vi "HIS.vi"(0 "System no.":i32=1 min=1 max=4 step=1, 2 "DeviceID":i32[](array[numeric]), 3 "Property":i32[](array[numeric]), 5 "error in":errorcluster, 6 "ItemID":i32[](array[numeric]), 10 "Value":string[](array[string])) -> (14 "Controller error":bool, 19 "error out":errorcluster)   [LabVIEW 2026]
doc: "This VI sets values for items of human interface devices (HID). The VI waits 100 ms and queries ERR?. Properties can be colors, the blink time of a LED, the frequency of a force-feed back function, display text etc. See controller user manual for details. Controller error is TRUE if selected system reports error code not equal to 0. \n\nC-884: Command is limited to set up to four DeviceIDs, ItemIDs, Properties and Values per call. ItemID must be of type \"LED\" which stands for hardware dependent output items or their properties."
panel:
  # "This vi sets values for items of human interface devices (HID). The VI waits 100 ms and queries ERR?.\nSee controller User Manual for details. Controller error is TRUE if selected system reports error code\nnot equal to 0."
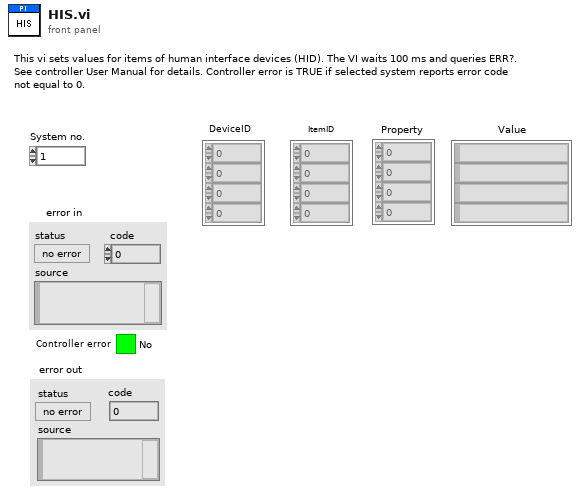
[diagram p1: front panel]
types:
  T1 = enum16{"Disable error check", "Force error check", "Use global settings"}
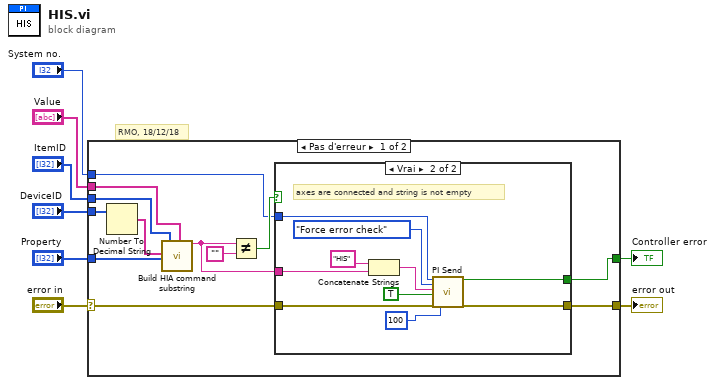
[diagram p0: block diagram]
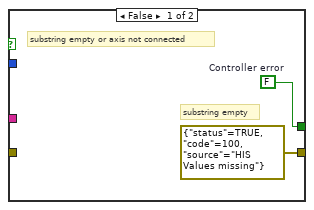
[diagram p2: hidden frame]
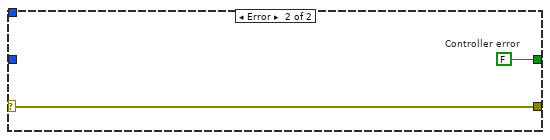
[diagram p3: hidden frame]
diagram:
  # "RMO, 18/12/18"
  n1 = case shown="Pas d'erreur" "error in" {
    selector: "error in" -> [w10 w34]
    tunnel: [w20 w34] -> w8
    tunnel: "Property" -> [w17 _]
    tunnel: "System no." -> [w14 _]
    tunnel: "DeviceID" -> [w13 _]
    tunnel: "ItemID" -> [w16 _]
    tunnel: "Value" -> [w11 _]
    tunnel: [w9 w33] -> w1
    frame No Error {
      n2 = Number To Decimal String(number=w13) -> (decimal integer string=w12:string[])  [unwired: 1 out]
      n3 = call "Build HIA command substring.vi"("Axes to set"=w12, "DeviceID"=w17, "Function"=w16, "DeviceAxis"=w11) -> ("HIA command substring"=w18:string)  [unwired: 1 in, 14 out]
      n4 = Not Equal?(x=w18, y="") -> (x != y?=w15:bool)
      n5 = case shown="Vrai" w15 {
        tunnel: w18 -> [_ w31]
        tunnel: [errorcluster {"status"=TRUE, "code"=100, "source"="HIS Values missing"} ("error out") w25] -> w20
        tunnel: w10 -> [_ w28]
        tunnel: w14 -> [_ w27]
        tunnel: [w21 w23] -> w9
        frame False {
          w21 = FALSE  # Controller error
          # "substring empty"
          # "substring empty or axis not connected"
        }
        frame True {
          # "axes are connected and string is not empty"
          n6 = Concatenate Strings("HIS", w31) -> (w29:string)
          n7 = call "PI Send.vi"("System no."=w27, "Error check settings"=T1."Force error check", "String to send"=w29, "Attach termination char.?"=TRUE ("Attach Linefeed?"), "error in"=w28, "Delay before error check (ms)"=u32 100 ("milliseconds to wait")) -> ("Controller error"=w23:bool, "error out"=w25:errorcluster)  [unwired: 12 out]
        }
      }
    }
    frame Error {
      w33 = FALSE  # Controller error
    }
  }
  "error out" <- w8
  "Controller error" <- w1
